vi "Sub_SharpSensor.vi"() -> (2 "links hinten":dbl, 3 "rechts hinten":dbl, 5 "schräg links":dbl, 6 "schräg rechts":dbl, 7 "links vorne":dbl, 8 "rechts vorne":dbl, 9 "gerade links":dbl, 10 "gerade rechts":dbl)   [LabVIEW 2016]
uses:
  <vilib>/myRIO/Instrument Drivers/Onboard IO/AI/typedefs/AI Reference.ctl
  <vilib>/myRIO/Common/Instrument Driver Framework/Utilities/typedefs/myRIO Generic Hardware Reference.ctl
  <vilib>/myRIO/Common/Instrument Driver Framework/Utilities/typedefs/Hardware Version Enum.ctl
  <vilib>/myRIO/Common/Instrument Driver Framework/Utilities/typedefs/myRIO v1.0 Reference.ctl
  <vilib>/myRIO/Common/Instrument Driver Framework/Utilities/typedefs/Generic FPGA Reference.ctl
  <vilib>/myRIO/Common/Instrument Driver Framework/myRIO v1.0/AI/typedefs/AI Channels List.ctl
  <vilib>/myRIO/Common/Instrument Driver Framework/myRIO v1.0/AI/typedefs/AI Channels Enum.ctl
  <vilib>/myRIO/Common/Instrument Driver Framework/Utilities/typedefs/Analog Scaling Constants List.ctl
  <vilib>/myRIO/Common/Instrument Driver Framework/Utilities/typedefs/Analog Scaling Constants.ctl
  <vilib>/userdefined/High Color/nirio_resource_hc.ctl
  <vilib>/myRIO/Common/Instrument Driver Framework/Utilities/vis/Is FPGA Ref Available.vi
  <vilib>/myRIO/Common/Instrument Driver Framework/myRIO v1.0/AI/vis/myRIO v1.1 Open AI.vi
  <vilib>/myRIO/Instrument Drivers/Onboard IO/AI/vis/Read.vi
  <vilib>/myRIO/Common/Instrument Driver Framework/Utilities/vis/Validate Channels.vi
  <vilib>/myRIO/Common/Instrument Driver Framework/myRIO v1.0/AI/vis/myRIO v1.0 Reserve AI.vi
  <vilib>/myRIO/Common/Instrument Driver Framework/myRIO v1.0/AI/vis/myRIO v1.0 Build MUX Configuration AI.vi
  <vilib>/myRIO/Common/Instrument Driver Framework/myRIO v1.0/Resource Manager/vis/myRIO v1.0 Reserve Channel List.vi
  <vilib>/myRIO/Common/Instrument Driver Framework/myRIO v1.0/Resource Manager/vis/myRIO v1.0 Reserve Channel.vi
  <vilib>/myRIO/Common/Instrument Driver Framework/myRIO v1.0/Resource Manager/vis/myRIO v1.0 Unreserve Channel.vi
  <vilib>/myRIO/Common/Instrument Driver Framework/myRIO v1.0/Resource Manager/vis/myRIO v1.0 Build Mutex Name.vi
  <vilib>/Utility/VariantDataType/GetNumericInfo.vi
  <vilib>/Utility/error.llb/Error Cluster From Error Code.vi
  <vilib>/myRIO/Common/Instrument Driver Framework/myRIO v1.0/myRIO v1.1 Open.vi
  <vilib>/myRIO/Common/Instrument Driver Framework/myRIO v1.0/AI/vis/myRIO v1.0 Get Scaling Constants AI.vi
  <vilib>/myRIO/Common/Instrument Driver Framework/Utilities/vis/IO Manager.vi
  <vilib>/myRIO/Common/Instrument Driver Framework/Utilities/vis/Configuration Manager.vi
  <vilib>/myRIO/Common/Instrument Driver Framework/myRIO v1.0/myRIO v1.0 Close.vi
  <vilib>/myRIO/Common/Instrument Driver Framework/myRIO v1.0/AI/vis/myRIO v1.0 Read AI.vi
  <vilib>/myRIO/Express VI/Onboard IO/AI/AI Express VI.xnode
  <vilib>/myRIO/Instrument Drivers/Onboard IO/AI/vis/myRIO AI Open.xnode
  <vilib>/myRIO/Instrument Drivers/Onboard IO/AI/AI.lvlib
panel:
  out "B/AI3 (Pin 9)":dbl=2.131347438
  out "A/AI3 (Pin 9)":dbl=2.131347438
  out "A/AI1 (Pin 5)":dbl=2.131347438
  out "A/AI0 (Pin 3)":dbl=2.131347438
  in  "rechts hinten":cluster{"a":dbl, " b":dbl, "c ":dbl}={"a"=10.03, " b"=-0.2533, "c "=1.001}
  out "B/AI0 (Pin 3) 8":dbl=2.131347438
  in  "links hinten":cluster{"a":dbl, " b":dbl, "c ":dbl}={"a"=10.03, " b"=-0.2533, "c "=1.001}
  in  "links schräg vorne":cluster{"a":dbl, " b":dbl, "c ":dbl}={"a"=13.06, " b"=0.7446, "c "=0.6199}
  in  "links gerade vorne":cluster{"a":dbl, " b":dbl, "c ":dbl}={"a"=13.66, " b"=3.318, "c "=0.2837}
  in  "rechts gerade vorne":cluster{"a":dbl, " b":dbl, "c ":dbl}={"a"=13.66, " b"=3.318, "c "=0.2837}
  out "B/AI1 (Pin 5)":dbl=2.131347438
  in  "rechts schräg vorne":cluster{"a":dbl, " b":dbl, "c ":dbl}={"a"=13.06, " b"=0.7446, "c "=0.6199}
  in  "rechts vorne":cluster{"a":dbl, " b":dbl, "c ":dbl}={"a"=10.03, " b"=-0.2533, "c "=1.001}
  out "A/AI2 (Pin 7)":dbl=2.131347438
  in  "links vorne":cluster{"a":dbl, " b":dbl, "c ":dbl}={"a"=10.03, " b"=-0.2533, "c "=1.001}
  out "B/AI2 (Pin 7)":dbl=2.131347438
  # "4-30\na: 10.03\nb:-0.2533\nc: 1.001"
  # "10-70\na: 13.06\nb: 0.7446\nc: 0.6199"
  # "20-150\na: 13.66\nb: 3.318\nc: 0.2837"
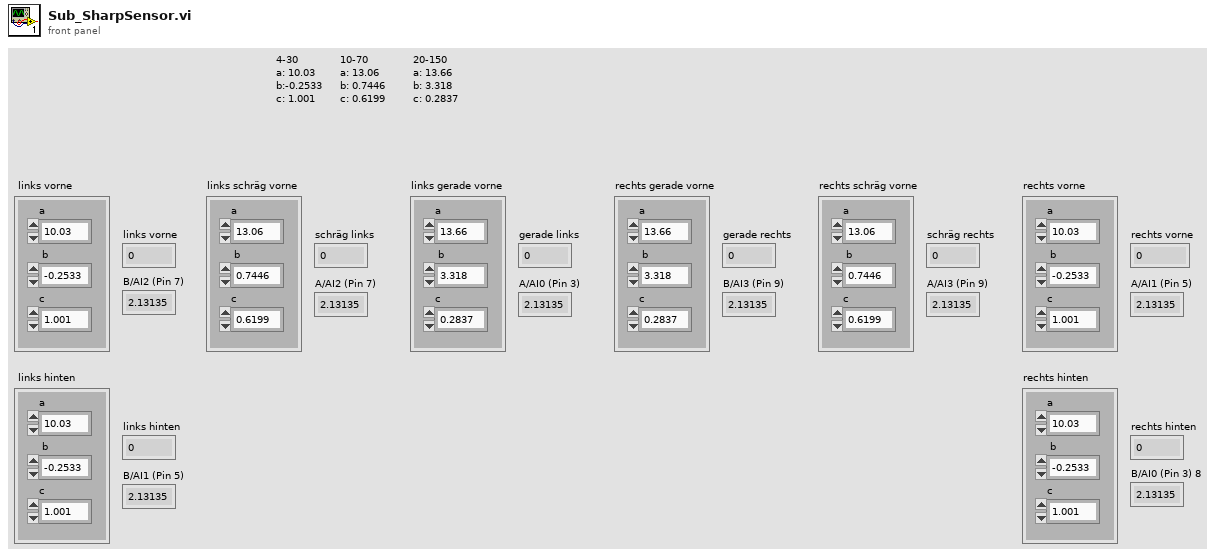
[diagram p1: front panel]
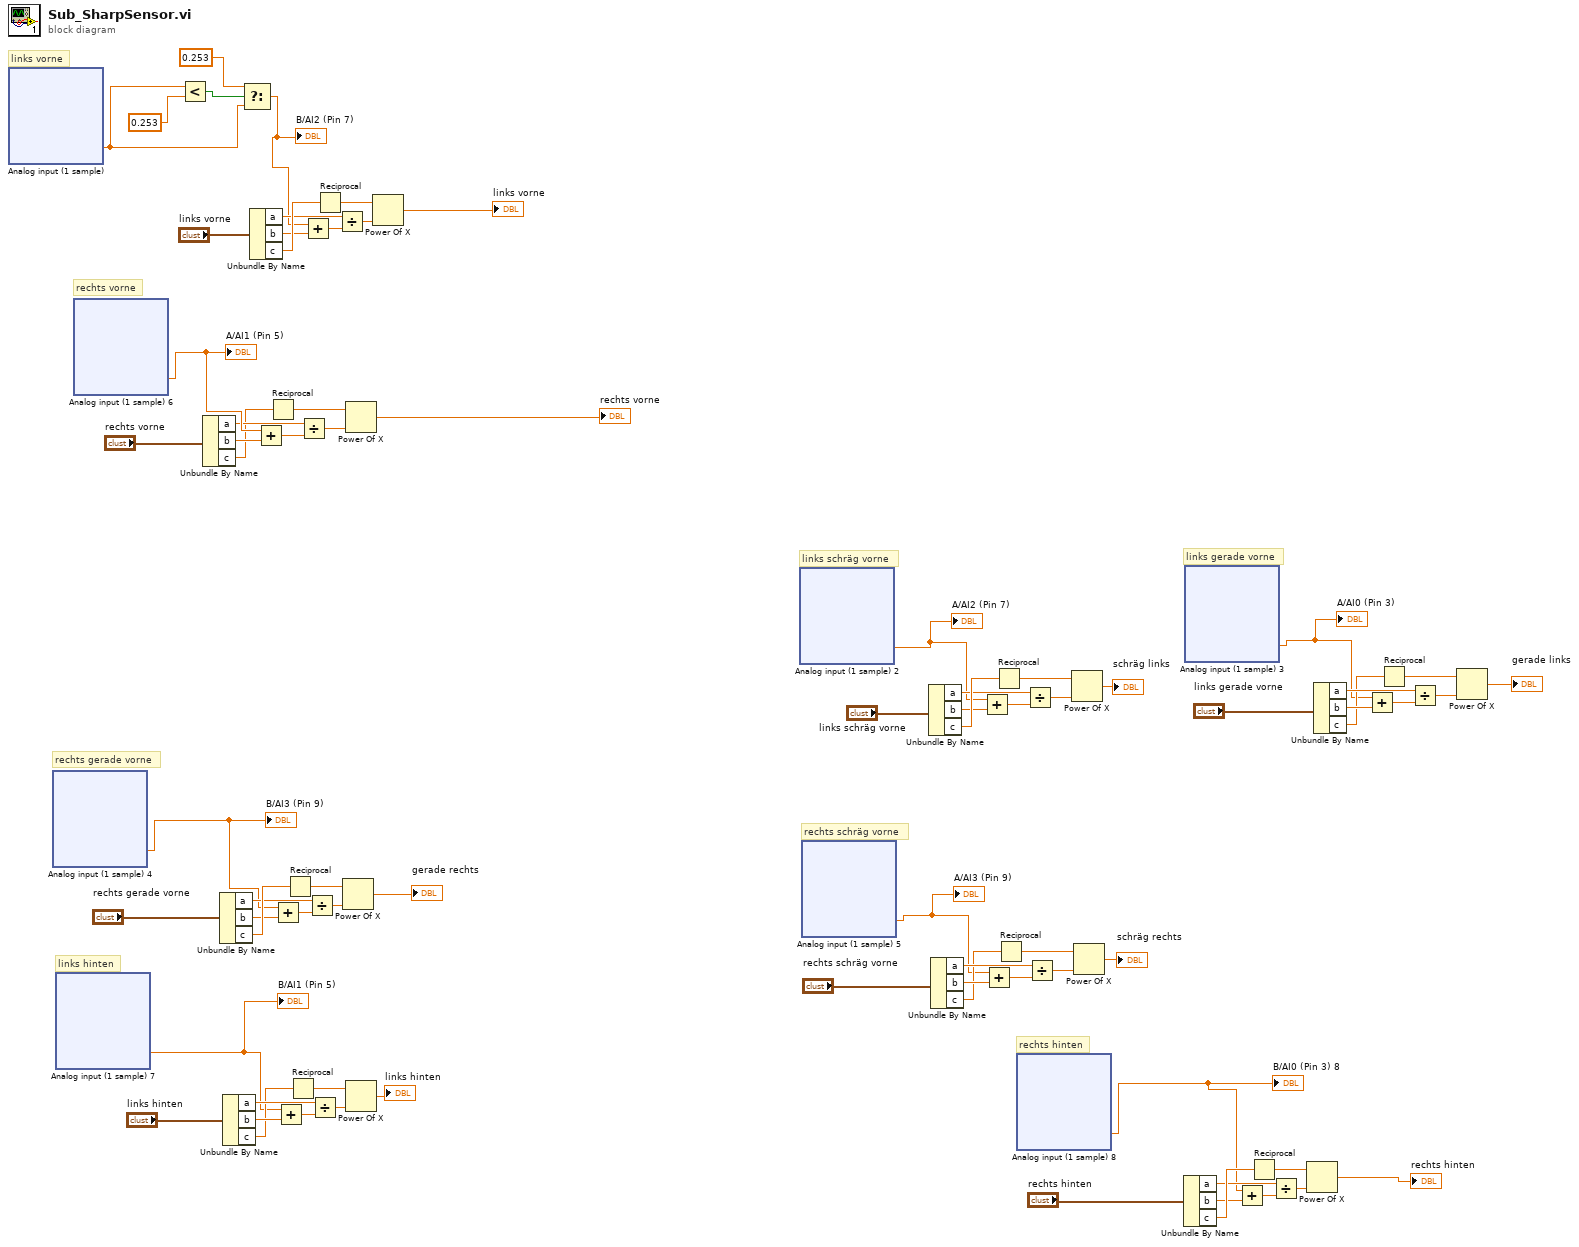
[diagram p0: block diagram]
diagram:
  # "rechts vorne"
  # "links vorne"
  # "rechts hinten"
  # "links hinten"
  # "rechts gerade vorne"
  # "rechts schräg vorne"
  # "links gerade vorne"
  # "links schräg vorne"
  n1 = xnode "Analog input (1 sample)"() -> ("B/AI2 (Pin 7)"=w3:dbl)  [unwired: 1 in, 1 out]
  n2 = xnode "Analog input (1 sample) 4"() -> ("A/AI1 (Pin 5)"=w24:dbl)  [unwired: 1 in, 1 out]
  "B/AI3 (Pin 9)" <- w24
  n3 = xnode "Analog input (1 sample) 7"() -> ("B/AI1 (Pin 5)"=w35:dbl)  [unwired: 1 in, 1 out]
  "B/AI1 (Pin 5)" <- w35
  n4 = xnode "Analog input (1 sample) 6"() -> ("B/AI3 (Pin 9)"=w22:dbl)  [unwired: 1 in, 1 out]
  "A/AI1 (Pin 5)" <- w22
  n5 = Less?(x=w3, y=0.253) -> (x < y?=w5:bool)
  n6 = Unbundle By Name("rechts vorne") -> ("a"=w20:dbl, "b"=w19:dbl, "c"=w16:dbl)
  n7 = Unbundle By Name("rechts gerade vorne") -> ("a"=w47:dbl, "b"=w48:dbl, "c"=w51:dbl)
  n8 = Unbundle By Name("links hinten") -> ("a"=w43:dbl, "b"=w42:dbl, "c"=w39:dbl)
  n9 = Select(t=0.253, s=w5, f=w3) -> (s? t:f=w2:dbl)
  "B/AI2 (Pin 7)" <- w2
  n10 = Unbundle By Name("links vorne") -> ("a"=w8:dbl, "b"=w9:dbl, "c"=w12:dbl)
  n11 = Add(x=w22, y=w19) -> (x+y=w18:dbl)
  n12 = Reciprocal(x=w16) -> (1/x=w15:dbl)
  n13 = Add(x=w24, y=w48) -> (x+y=w49:dbl)
  n14 = Add(x=w35, y=w42) -> (x+y=w41:dbl)
  n15 = Reciprocal(x=w51) -> (1/x=w52:dbl)
  n16 = Reciprocal(x=w39) -> (1/x=w38:dbl)
  n17 = Divide(x=w20, y=w18) -> (x/y=w17:dbl)
  n18 = Add(x=w2, y=w9) -> (x+y=w10:dbl)
  n19 = Divide(x=w47, y=w49) -> (x/y=w50:dbl)
  n20 = Divide(x=w43, y=w41) -> (x/y=w40:dbl)
  n21 = Reciprocal(x=w12) -> (1/x=w13:dbl)
  n22 = Divide(x=w8, y=w10) -> (x/y=w11:dbl)
  n23 = Power Of X(1:w50, 2:w52) -> (0:→"gerade rechts":dbl)
  n24 = Power Of X(1:w17, 2:w15) -> (0:→"rechts vorne":dbl)
  n25 = Power Of X(1:w40, 2:w38) -> (0:→"links hinten":dbl)
  n26 = Power Of X(1:w11, 2:w13) -> (0:→"links vorne":dbl)
  n27 = xnode "Analog input (1 sample) 2"() -> ("A/AI2 (Pin 7)"=w60:dbl)  [unwired: 1 in, 1 out]
  "A/AI2 (Pin 7)" <- w60
  n28 = xnode "Analog input (1 sample) 5"() -> ("A/AI3 (Pin 9)"=w45:dbl)  [unwired: 1 in, 1 out]
  "A/AI3 (Pin 9)" <- w45
  n29 = Unbundle By Name("links schräg vorne") -> ("a"=w71:dbl, "b"=w72:dbl, "c"=w75:dbl)
  n30 = Unbundle By Name("rechts schräg vorne") -> ("a"=w58:dbl, "b"=w57:dbl, "c"=w54:dbl)
  n31 = Add(x=w60, y=w72) -> (x+y=w73:dbl)
  n32 = Add(x=w45, y=w57) -> (x+y=w56:dbl)
  n33 = Reciprocal(x=w75) -> (1/x=w76:dbl)
  n34 = Reciprocal(x=w54) -> (1/x=w53:dbl)
  n35 = xnode "Analog input (1 sample) 8"() -> ("B/AI0 (Pin 3)"=w23:dbl)  [unwired: 1 in, 1 out]
  "B/AI0 (Pin 3) 8" <- w23
  n36 = Divide(x=w71, y=w73) -> (x/y=w74:dbl)
  n37 = Divide(x=w58, y=w56) -> (x/y=w55:dbl)
  n38 = Power Of X(1:w74, 2:w76) -> (0:→"schräg links":dbl)
  n39 = Power Of X(1:w55, 2:w53) -> (0:→"schräg rechts":dbl)
  n40 = Unbundle By Name("rechts hinten") -> ("a"=w28:dbl, "b"=w29:dbl, "c"=w32:dbl)
  n41 = xnode "Analog input (1 sample) 3"() -> ("A/AI0 (Pin 3)"=w59:dbl)  [unwired: 1 in, 1 out]
  "A/AI0 (Pin 3)" <- w59
  n42 = Add(x=w23, y=w29) -> (x+y=w30:dbl)
  n43 = Reciprocal(x=w32) -> (1/x=w33:dbl)
  n44 = Divide(x=w28, y=w30) -> (x/y=w31:dbl)
  n45 = Power Of X(1:w31, 2:w33) -> (0:→"rechts hinten":dbl)
  n46 = Unbundle By Name("links gerade vorne") -> ("a"=w69:dbl, "b"=w68:dbl, "c"=w65:dbl)
  n47 = Add(x=w59, y=w68) -> (x+y=w67:dbl)
  n48 = Reciprocal(x=w65) -> (1/x=w64:dbl)
  n49 = Divide(x=w69, y=w67) -> (x/y=w66:dbl)
  n50 = Power Of X(1:w66, 2:w64) -> (0:→"gerade links":dbl)
